vi "GetParam.vi"(8 "error in (no error)":errorcluster caption="entrée d'erreur (pas d'erreur)", 11 "IterativeImputer.lvclass":refnum<class "IterativeImputer.lvclass">) -> (0 "error out":errorcluster caption="sortie d'erreur", 2 "IterativeImputer":T1={"estimator"="None", "missing_values"="nan", "sample_posterior"=FALSE, "max_iter"=10, "tol"=0.001, "n_nearest_features"=-1, "initial_strategy"="mean", "imputation_order"="ascending", "skip_complete"=FALSE, "min_value"=["None"], "max_value"=["None"], "verbose"=0, "random_state"=-1, "add_indicator"=FALSE} {"random_state" min=-1; "n_nearest_features" min=-1}, 3 "IterativeImputer.lvclass":refnum<class "IterativeImputer.lvclass">)   [LabVIEW 2020, in "IterativeImputer.lvclass"]
doc: "Get Parameters"
uses:
  IterativeImputer.lvclass
  IterativeImputer.lvclass/IterativeImputer.ctl
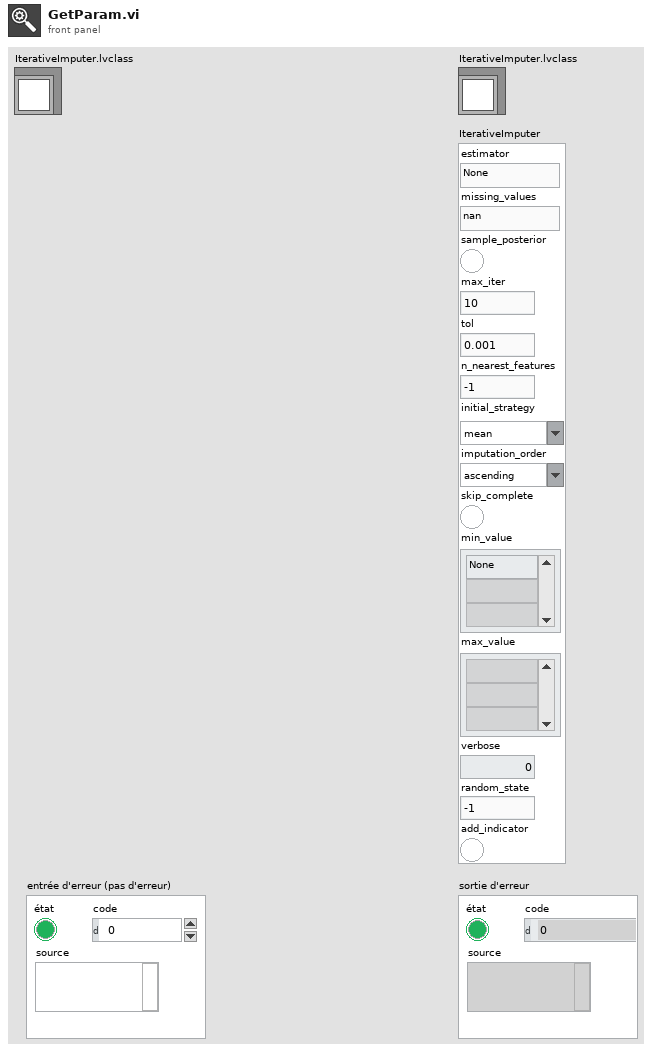
[diagram p1: front panel]
types:
  T1 = cluster{"estimator":string, "missing_values":string, "sample_posterior":bool, "max_iter":i32, "tol":dbl, "n_nearest_features":i32, "initial_strategy":string, "imputation_order":string, "skip_complete":bool, "min_value":string[], "max_value":string[], "verbose":i32, "random_state":i32, "add_indicator":bool}
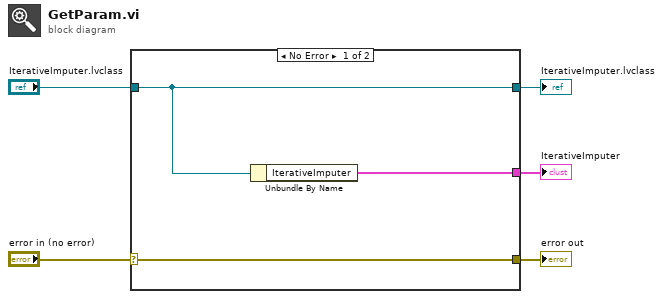
[diagram p0: block diagram]
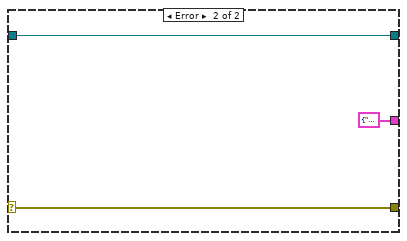
[diagram p2: hidden frame]
diagram:
  n1 = case shown="No Error" "error in (no error)" {
    selector: "error in (no error)" -> [w8 w10]
    tunnel: [w8 w10] -> w4
    tunnel: [w7 w11] -> w2
    tunnel: "IterativeImputer.lvclass" -> [w7 w11]
    tunnel: [w6 T1 {"estimator"="", "missing_values"="", "sample_posterior"=FALSE, "max_iter"=0, "tol"=0.0, "n_nearest_features"=0, "initial_strategy"="", "imputation_order"="", "skip_complete"=FALSE, "min_value"=[], "max_value"=[], "verbose"=0, "random_state"=0, "add_indicator"=FALSE} ("IterativeImputer")] -> w1
    frame No Error {
      n2 = Unbundle By Name(w7) -> ("IterativeImputer"=w6:T1)
    }
    frame Error {
    }
  }
  "error out" <- w4
  "IterativeImputer.lvclass" <- w2
  "IterativeImputer" <- w1
